vi "Start Phase.vi"(4 "array":string[][](array[string]), 8 "error in (no error)":errorcluster, 10 "index (row)":u16, 11 "Programming Logicv2 in":refnum<class "Programming Logicv2.lvclass">) -> (0 "error out":errorcluster, 1 "Speed":string, 2 "Direction":string, 3 "Programming Logicv2 out":refnum<class "Programming Logicv2.lvclass">, 5 "Temp":string, 7 "Time":string)   [LabVIEW 2014, in "Main Libraryv2.lvlib" / "Programming Logicv2.lvclass"]
uses:
  Programming Logicv2.lvclass
  Control/Main Libraryv2.lvlib
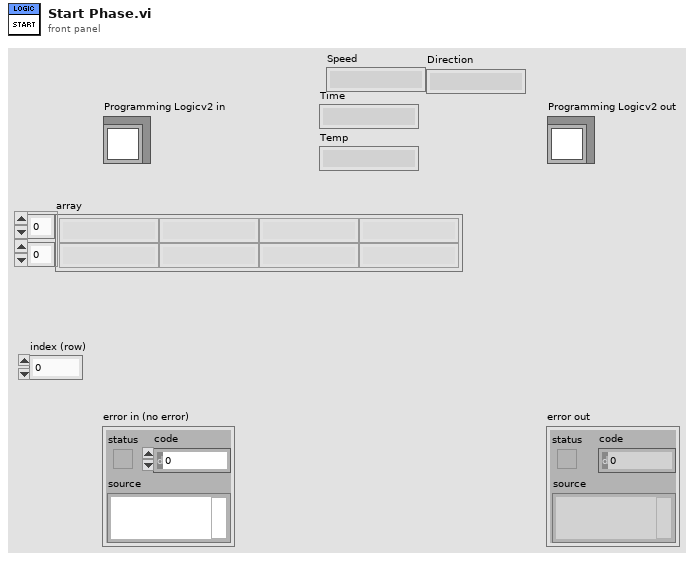
[diagram p1: front panel]
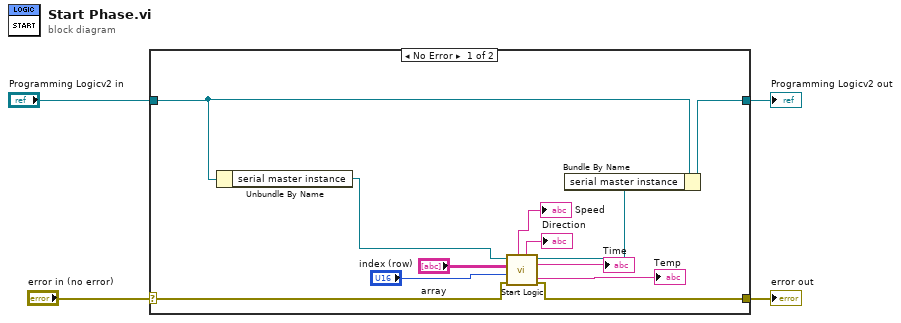
[diagram p0: block diagram]
diagram:
  n1 = case shown="No Error" "error in (no error)" {
    selector: "error in (no error)" -> [w5 w18]
    tunnel: [w6 w18] -> w3
    tunnel: [w16 w17] -> w1
    tunnel: "Programming Logicv2 in" -> [w15 w17]
    frame No Error {
      n2 = Unbundle By Name(w15) -> ("serial master instance"=w9:refnum<class "Modbus Master.lvclass">)
      n3 = call "Start Logic.vi"("error in"=w5, "index (row)"="index (row)", "array"="array", "Modbus master in"=w9) -> ("error out"=w6:errorcluster, "Modbus master out"=w8:refnum<class "Modbus Master.lvclass">, "Time"=→"Time":string, "Direction"=→"Direction":string, "Temp"=→"Temp":string, "Speed"=→"Speed":string)  [unwired: 2 in]
      n4 = Bundle By Name(cluster=w15, "serial master instance"=w8) -> (w16:refnum<class "Programming Logicv2.lvclass">)
    }
    frame Error {
    }
  }
  "error out" <- w3
  "Programming Logicv2 out" <- w1
